vi "LimitTest.vi"(5 "RX?":bool=TRUE, 7 "AlarmCfg":T1 {"ErrsAndWarns" scale=0.0..10.0}, 10 "Source":string, 11 "Data":dbl) -> (3 "ErrorStatus":T2)   [LabVIEW 2018]
uses:
  Controls/Clusts/ErrorStatus.ctl
  Controls/Clusts/AlarmThresh_OneChan.ctl
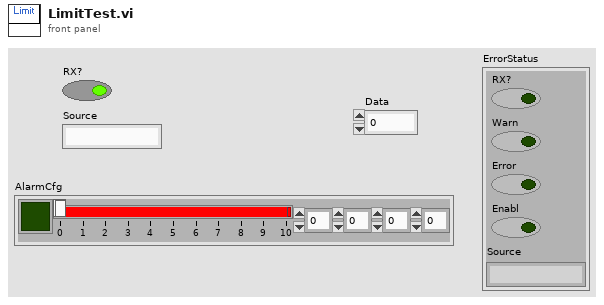
[diagram p1: front panel]
types:
  T1 = typedef "AlarmThresh_OneChan.ctl" = cluster{"Enbl":bool, "ErrsAndWarns":cluster{dbl, dbl, dbl, dbl}}
  T2 = typedef "ErrorStatus.ctl" = cluster{"RX?":bool, "Warn":bool, "Error":bool, "Enabl":bool, "Source":string}
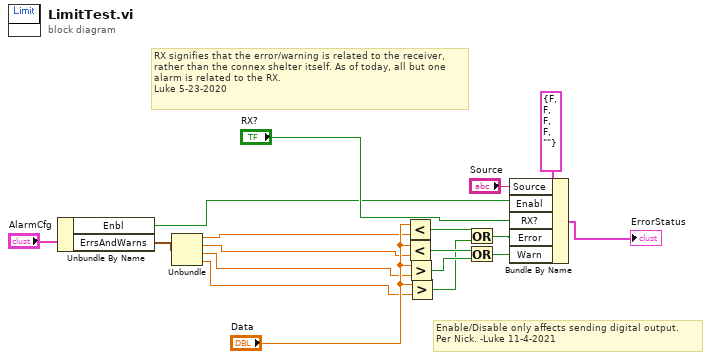
[diagram p0: block diagram]
diagram:
  # "Enable/Disable only affects sending digital output.\nPer Nick. -Luke 11-4-2021"
  # "RX signifies that the error/warning is related to the receiver,\nrather than the connex shelter itself. As of today, all but one\nalarm is related to the RX.\nLuke 5-23-2020"
  n1 = Unbundle By Name("AlarmCfg") -> ("Enbl"=w12:bool, "ErrsAndWarns"=w15:cluster{dbl, dbl, dbl, dbl})
  n2 = Unbundle(w15) -> (w11:dbl, w10:dbl, w9:dbl, w8:dbl)
  n3 = Less?(x="Data", y=w11) -> (x < y?=w2:bool)
  n4 = Less?(x="Data", y=w10) -> (x < y?=w4:bool)
  n5 = Greater?(x="Data", y=w9) -> (0:w5:bool)
  n6 = Greater?(x="Data", y=w8) -> (0:w3:bool)
  n7 = Or(x=w2, y=w3) -> (x .or. y?=w6:bool)
  n8 = Or(x=w4, y=w5) -> (x .or. y?=w7:bool)
  n9 = Bundle By Name(cluster=T2 {"RX?"=FALSE, "Warn"=FALSE, "Error"=FALSE, "Enabl"=FALSE, "Source"=""}, "Source"="Source", "Enabl"=w12, "RX?"="RX?", "Error"=w6, "Warn"=w7) -> (→"ErrorStatus":T2)
